vi "NewSerialPort.vi"(6 "timeout (10sec)":u32=500, 7 "termination char\n(0xA = '\\n' = LF)":u8, 8 "BaudRate":string, 9 "Enable":bool, 10 "Enable Termination\nChar (T)":bool=TRUE, 11 "COMPort":string) -> (0 "error out":errorcluster, 3 "VISA Out":refnum<visa-resource-name>)   [LabVIEW 2017]
uses:
  <vilib>/Instr/_visa.llb/VISA Configure Serial Port (Instr).vi
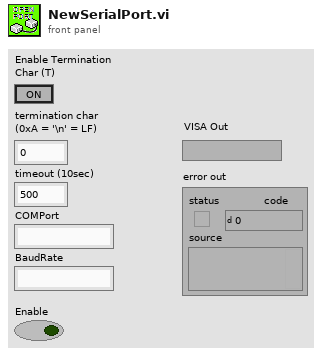
[diagram p1: front panel]
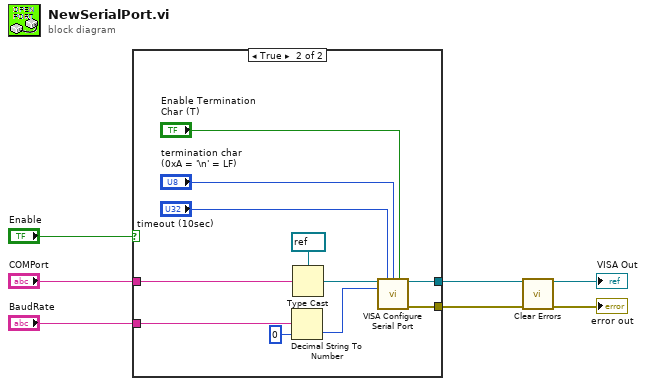
[diagram p0: block diagram]
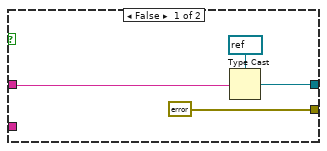
[diagram p2: hidden frame]
diagram:
  n1 = case shown="True" "Enable" {
    tunnel: "COMPort" -> [w7 w15]
    tunnel: "BaudRate" -> [_ w14]
    tunnel: [w8 w13] -> w4
    tunnel: [errorcluster {"status"=FALSE, "code"=0, "source"=""} ("error out") w12] -> w2
    frame False {
      n2 = Type Cast(type=refnum<visa-resource-name> refnum ("VISA resource name"), x=w7) -> (*(type *) &x=w8:refnum<visa-resource-name>)
    }
    frame True {
      n3 = Decimal String To Number(string=w14, default (0L)=u32 0 ("default (0 I32)")) -> (number=w16:u32)  [unwired: 1 in, 1 out]
      n4 = Type Cast(type=refnum<visa-resource-name> refnum ("VISA resource name"), x=w15) -> (*(type *) &x=w19:refnum<visa-resource-name>)
      n5 = call-poly "VISA Configure Serial Port"("VISA resource name"=w19, "timeout (10sec)"="timeout (10sec)", "termination char\n(0xA = '\\n' = LF)"="termination char\n(0xA = '\\n' = LF)", "Enable Termination\nChar (T)"="Enable Termination\nChar (T)", "baud rate (9600)"=w16) -> ("VISA resource name out"=w13:refnum<visa-resource-name>, "error out"=w12:errorcluster)  [unwired: 9 in]
    }
  }
  "VISA Out" <- w4
  n6 = call <vilib>:"Clear Errors.vi"("error in (no error)"=w2) -> ("error out"=→"error out":errorcluster)  [unwired: 5 in, 1 out]
